vi "ClsExecCommand.vi"(8 "error in (no error)":errorcluster, 10 "Command In":string, 11 "Connection In":u32) -> (0 "error out":errorcluster, 2 "Command Response":string, 3 "Connection Out":u32)   [LabVIEW 2015]
doc: "Exec Command:\n\nUse this VI to execute a command(SOD or SODX is not allowed here. Use Set Output Signals subVI to set signal IDs for output). This function will send client specified command to device. It flushes all the received sample, send command and wait for the response. In another word, it uses the blocking mode. If the response has not come in 15 seconds for $DRK and $WHT command, 5 seconds for all the other commands, it will stop waiting and report error.\n\nConnection In[Input]: the connection handle which is initially created by Open Connection subVI.\n\nCommand In[Input]: String for command which should begin with \"$\". For example, \"$NOP 3\" \"$AVD ?\" \"$SHZ 1000\", etc..\n\nCommand Response[Output]: String of command response.\n\nConnection Out[Output]: the connection handle output which could be used for next subVI refering to the same connection."
uses:
  <vilib>/Utility/importsl/GetValueByPointer/datatype.ctl
  <vilib>/Utility/importsl/GetValueByPointer/GetValueByPointer.xnode
  lvimptsl.dll
  dependent dlls/CHRocodileDLL.dll
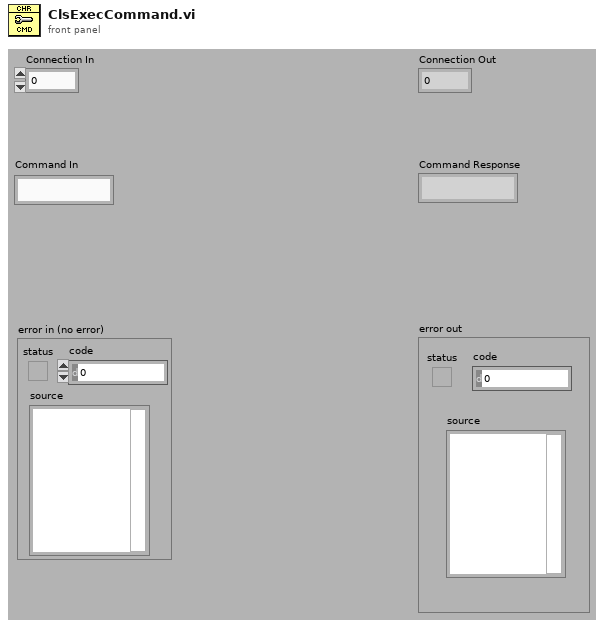
[diagram p1: front panel]
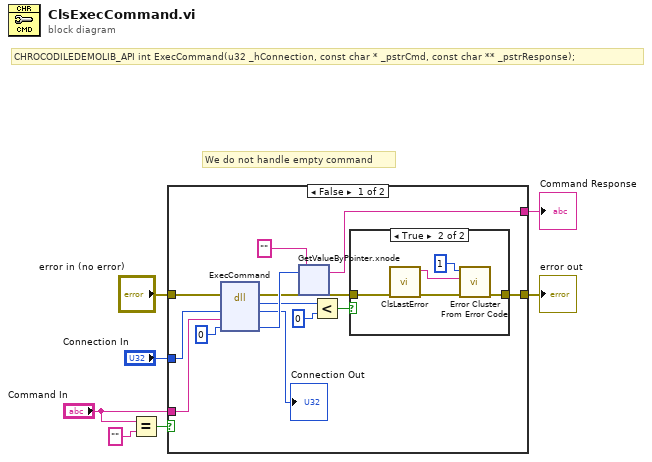
[diagram p0: block diagram]
diagram:
  # "We do not handle empty command"
  # "CHROCODILEDEMOLIB_API int ExecCommand(u32 _hConnection, const char * _pstrCmd, const char ** _pstrResponse);"
  n1 = Equal?(x="Command In", y="") -> (x = y?=w1:bool)
  n2 = case shown="False" w1 {
    tunnel: "Connection In" -> [w21 _]
    tunnel: "error in (no error)" -> [w18 w36]
    tunnel: [w15 w37] -> w5
    tunnel: [w14 w36] -> w4
    tunnel: "Command In" -> [w8 w37]
    frame False {
      n3 = dll-call lib="C:/Users/privat/Documents/ADP-SLA/Drop Impact Teststand/dependent dlls/CHRocodileDLL.*" fn="ExecCommand"(error in=w18, "_hConnection"=w21, "_pstrCmd"=w8, "_pstrResponse"=i64 0) -> (error out=w17:errorcluster, "return type"=w11:i32, "_hConnection"=→"Connection Out":u32, "_pstrResponse"=w19:i64)  [unwired: 3 in, 1 out]
      n4 = xnode "GetValueByPointer.xnode"("Pointer"=w19, "InputType"="" ("_pstrCmd 2"), "ErrorIn"=w17) -> ("Output"=w15:string, "ErrorOut"=w9:errorcluster)  [unwired: 1 in]
      n5 = Less?(x=w11, y=0) -> (x < y?=w12:bool)
      n6 = case shown="True" w12 {
        tunnel: [w22 w23] -> w14
        tunnel: w9 -> [w22 w27]
        frame False {
        }
        frame True {
          n7 = call "ClsLastError.vi"("error in (no error)"=w27) -> ("error out"=w25:errorcluster, "Error Message"=w26:string)  [unwired: 9 in]
          n8 = call <vilib>:"Error Cluster From Error Code.vi"("error in (no error)"=w25, "error message (\"\")"=w26, "error code (0)"=1) -> ("error out"=w23:errorcluster)  [unwired: 6 in]
        }
      }
    }
    frame True {
    }
  }
  "Command Response" <- w5
  "error out" <- w4
